vi "test IAM.vi"() -> ()   [LabVIEW 2015]
uses:
  Policy.ctl
  Core/HTTP Request/AWS Credentials.ctl
  IAM Session/IAM Session.lvclass
  Core/HTTP Request/HTTP Request.lvclass
  NI_AWS_IAM.lvlib
panel:
  out "Policies":T1[](array[typedef])
  out "error out":errorcluster
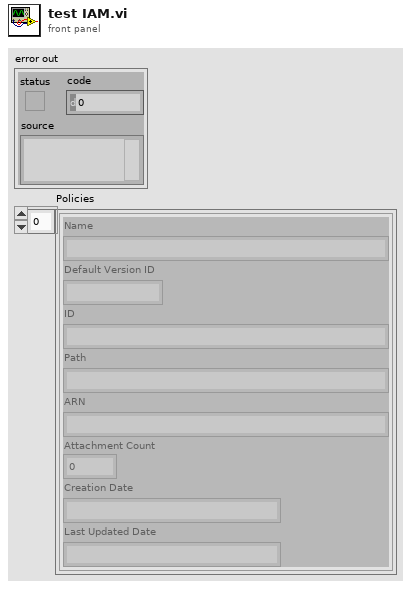
[diagram p1: front panel]
types:
  T1 = typedef "NI_AWS_IAM.lvlib/Policy.ctl" = cluster{"Name":string, "Default Version ID":string, "ID":string, "Path":string, "ARN":string, "Attachment Count":i32, "Creation Date":string, "Last Updated Date":string}
  T2 = typedef "NI_AWS_Core.lvlib/HTTP Request.lvclass/AWS Credentials.ctl" = cluster{"Access Key":string, "Secret Key":string}
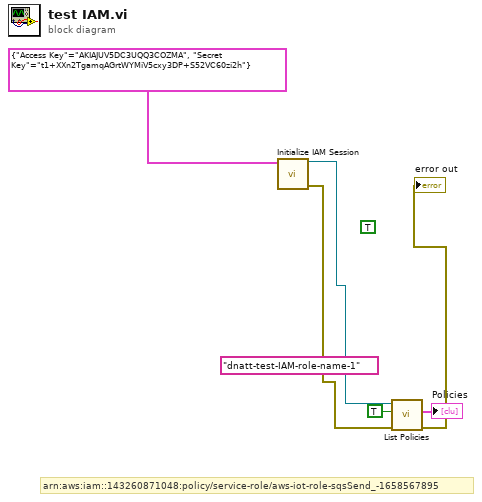
[diagram p0: block diagram]
diagram:
  (unwired) "dnatt-test-IAM-role-name-1" ("Role")
  (unwired) TRUE ("Only Attached")
  # "arn:aws:iam::143260871048:policy/service-role/aws-iot-role-sqsSend_-1658567895"
  n1 = call "Initialize IAM Session.vi"("AWS Credentials"=T2 {"Access Key"="AKIAJUV5DC3UQQ3COZMA", "Secret Key"="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"}) -> ("error out"=w5:errorcluster, "IAM Session"=w4:refnum<class "IAM Session.lvclass">)  [unwired: 9 in]
  n2 = call "List Policies.vi"("error in (no error)"=w5, "Only Attached"=TRUE, "IAM Session in"=w4) -> ("error out"=→"error out":errorcluster, "Policies"=→"Policies":T1[])  [unwired: 6 in, 1 out]
